vi "PH_PSDBController.set Status.vi"(0 "i ref in":refnum<vi>, 5 "error in":errorcluster) -> (14 "i ref out":refnum<vi>, 19 "error out":errorcluster)   [LabVIEW 2014, in "PH_PSDBController.lvlib"]
uses:
  PH_PSDBController.lvlib
  PH_StatusHandler/PH_StatusHandler.Status.ctl
  PH_PSDBWriter/PH_PSDBWriter.Data Status.ctl
  PH_PSDBWriter/PH_PSDBWriter.lvlib
  PH_StatusHandler/PH_StatusHandler.lvlib
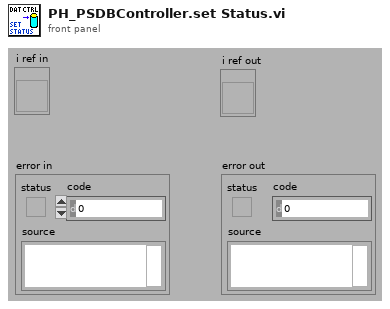
[diagram p1: front panel]
types:
  T1 = typedef "PH_PSDBWriter.lvlib/PH_PSDBWriter.Data Status.ctl" = i16
  T2 = typedef "PH_StatusHandler.lvlib/PH_StatusHandler.Status.ctl" = i16
  T3 = typedef "PH_PSDBController.lvlib/PH_PSDBController.i attribute.ctl" = cluster{"GUI Refs":cluster{"Data Status":refnum<vi>, "Current Shot ID":refnum<vi>, "active Subsystems":refnum<vi>, "Experiment Description":refnum<vi>, "Shot Comment":refnum<vi>, "Experiment":refnum<vi>, "Shottype":refnum<vi>, "Sequencer SM State":refnum<vi>, "Instances with Errors":refnum<vi>}, "Service ID Shot ID":i32, "Service ID wanted Subsystem":i32, "Data Status":T1, "Shotinformation":cluster{"Current Experiment ID":i32, "Current Shot Type":i32, "Current Comment":string}, "Data taking?":bool, "Service ID current Shottype":i32, "Service ID current Experiment":i32, "Service ID currentShot Comment":i32, "Service ID possible Shottypes":i32, "Service ID possible Experiments":i32, "possible Experiments":T4[], "possible Shottypes":T4[], "List":cluster{"Info":cluster{"Instance":string, "Data Status":T1}[], "GUI Ref":refnum<vi>, "Classname":string}[], "Subsystems Off?":cluster{"PHELIX_Beamline_fs_YLF_BL_Status":bool, "PHELIX_Beamline_ns_BL_Status":bool, "PHELIX_Beamline_PA_Input_BL_Status":bool, "PHELIX_Beamline_PA_MA_BL_Status":bool, "PHELIX_Beamline_MA_Z6_BL_Status":bool, "PHELIX_Beamline_MA_LB_BL_Status":bool, "PHELIX_Beamline_PA_LL_BL_Status":bool}, "PSDB Credentials":T5}
  T4 = typedef "PSDB.lvlib/PSDB_Info.ctl" = cluster{"Name":string, "Description":string, "ID":i32}
  T5 = typedef "PH_Common.lvlib/PH_Connection.PSDB Credentials.ctl" = cluster{"PW":string, "ID":string, "DS":string}
  T6 = cluster{"Info":cluster{"Instance":string, "Data Status":T1}[], "GUI Ref":refnum<vi>, "Classname":string}[]
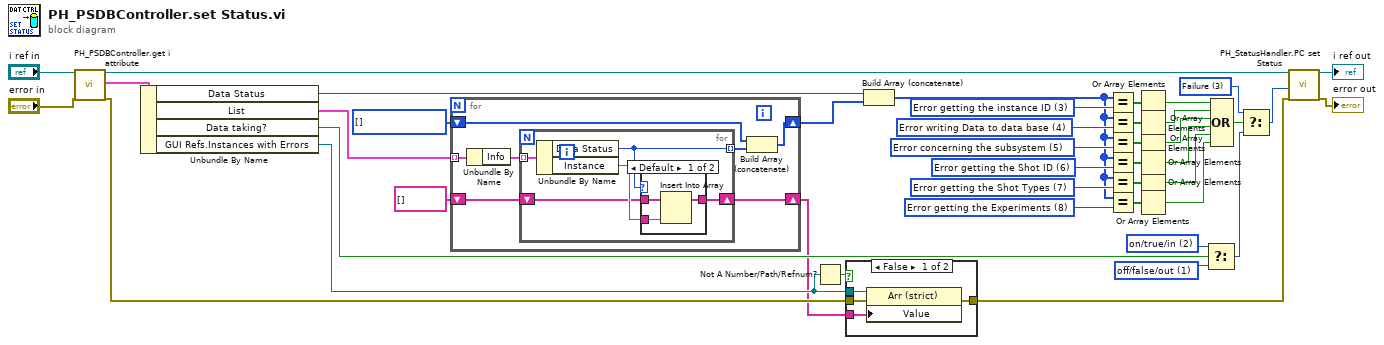
[diagram p0: block diagram]
diagram:
  w11 = T1[] [] items=["no info", "no Data collection", "no problem", "Error getting the instance ID", "Error writing Data to data base", "Error concerning the subsystem", "Error getting the Shot ID", "Error getting the Shot Types", "Error getting the Experiments", "Error verifying wanted Shottype", "Error verifying wanted Experiment"]
  w23 = T1 8 items=["no info", "no Data collection", "no problem", "Error getting the instance ID", "Error writing Data to data base", "Error concerning the subsystem", "Error getting the Shot ID", "Error getting the Shot Types", "Error getting the Experiments"] ("Data Status")
  w24 = T1 7 items=["no info", "no Data collection", "no problem", "Error getting the instance ID", "Error writing Data to data base", "Error concerning the subsystem", "Error getting the Shot ID", "Error getting the Shot Types", "Error getting the Experiments"] ("Data Status")
  w25 = T1 6 items=["no info", "no Data collection", "no problem", "Error getting the instance ID", "Error writing Data to data base", "Error concerning the subsystem", "Error getting the Shot ID", "Error getting the Shot Types", "Error getting the Experiments"] ("Data Status")
  w26 = T1 5 items=["no info", "no Data collection", "no problem", "Error getting the instance ID", "Error writing Data to data base", "Error concerning the subsystem", "Error getting the Shot ID", "Error getting the Shot Types", "Error getting the Experiments"] ("Data Status")
  w27 = T1 4 items=["no info", "no Data collection", "no problem", "Error getting the instance ID", "Error writing Data to data base", "Error concerning the subsystem", "Error getting the Shot ID", "Error getting the Shot Types", "Error getting the Experiments"] ("Data Status")
  w28 = T1 3 items=["no info", "no Data collection", "no problem", "Error getting the instance ID", "Error writing Data to data base", "Error concerning the subsystem", "Error getting the Shot ID", "Error getting the Shot Types", "Error getting the Experiments"] ("Data Status")
  w29 = T2 1 items=["no info", "off/false/out", "on/true/in", "Failure", "Alarm", "Status 1", "Status 2", "Status 3"] ("f")
  w30 = T2 2 items=["no info", "off/false/out", "on/true/in", "Failure", "Alarm", "Status 1", "Status 2", "Status 3"] ("Status")
  w36 = T2 3 items=["no info", "off/false/out", "on/true/in", "Failure", "Alarm", "Status 1", "Status 2", "Status 3"] ("Status")
  n1 = call "PH_PSDBController.get i attribute.vi"("i ref in"="i ref in", "error in (no error)"="error in") -> ("i ref out"=w2:refnum<vi>, "i attribute"=w40:T3, "error out"=w5:errorcluster)  [unwired: 15 in]
  n2 = Unbundle By Name(w40) -> ("Data Status"=w34:T1, "List"=w13:T6, "Data taking?"=w31:bool, "GUI Refs.Instances with Errors"=w7:refnum<vi>)
  n3 = for {
    tunnel: w13 -> [w49] mode=indexing
    shift-right: [w46] -> w12
    shift-left: w11 -> [w45]
    shift-right: [w44] -> w4
    shift-left: string[] [] -> [w43]
    n4 = Unbundle By Name(w49) -> ("Info"=w48:cluster{"Instance":string, "Data Status":T1}[])
    n5 = for {
      tunnel: w48 -> [w54] mode=indexing
      tunnel: [w53] -> w47 mode=indexing
      shift-right: [w51] -> w44
      shift-left: w43 -> [w50]
      n6 = Unbundle By Name(w54) -> ("Data Status"=w53:T1, "Instance"=w52:string)
      n7 = case shown="Default" w53 {
        tunnel: w52 -> [w57 _]
        tunnel: [w56 w58] -> w51
        tunnel: w50 -> [w55 w58]
        frame Default {
          n8 = Insert Into Array(array=w55, new element=w57) -> (w56:string[])  [unwired: 1 in]
        }
        frame 0..2 {
        }
      }
    }
    n9 = Build Array (concatenate)(w45, w47) -> (w46:T1[])
  }
  n10 = Not A Number/Path/Refnum?(number/path/refnum=w7) -> (NaN/Path/Refnum?=w9:bool)
  n11 = case shown="False" w9 {
    tunnel: w5 -> [w62 w63]
    tunnel: [w61 w63] -> w6
    tunnel: w7 -> [w60 _]
    tunnel: w4 -> [w59 _]
    frame False {
      n12 = property class="Arr (strict)"(reference=w60, error in=w62, "Value"=w59) -> (error out=w61:errorcluster)  [unwired: 1 out]
    }
    frame True {
    }
  }
  n13 = Build Array (concatenate)(w34, w12) -> (w22:T1[])
  n14 = Equal?(x=w22, y=w28) -> (x = y?=w33:bool[])
  n15 = Equal?(x=w22, y=w27) -> (x = y?=w38:bool[])
  n16 = Equal?(x=w22, y=w26) -> (x = y?=w21:bool[])
  n17 = Equal?(x=w22, y=w25) -> (x = y?=w20:bool[])
  n18 = Equal?(x=w22, y=w24) -> (x = y?=w19:bool[])
  n19 = Equal?(x=w22, y=w23) -> (x = y?=w18:bool[])
  n20 = Or Array Elements(Boolean array=w33) -> (logical OR=w32:bool)
  n21 = Or Array Elements(Boolean array=w38) -> (logical OR=w37:bool)
  n22 = Or Array Elements(Boolean array=w21) -> (logical OR=w17:bool)
  n23 = Or Array Elements(Boolean array=w20) -> (logical OR=w16:bool)
  n24 = Or Array Elements(Boolean array=w19) -> (logical OR=w15:bool)
  n25 = Or Array Elements(Boolean array=w18) -> (logical OR=w14:bool)
  n26 = Select(t=w30, s=w31, f=w29) -> (s? t:f=w10:T2)
  n27 = Compound Arithmetic op=OR(w32, w37, w17, w16, w15, w14) -> (w39:bool)
  n28 = Select(t=w36, s=w39, f=w10) -> (s? t:f=w35:T2)
  n29 = call "PH_StatusHandler.PC set Status.vi"("i ref in"=w2, "Status"=w35, "error in (no error)"=w6) -> ("i ref out"=→"i ref out":refnum<vi>, "error out"=→"error out":errorcluster)  [unwired: 15 in]
